vi "destroy_lookup.vi"(8 "error in (no error)":errorcluster, 11 "Mapped Lookup in":refnum<class "Mapped Lookup.lvclass">) -> (0 "error out":errorcluster)   [LabVIEW 2019, in "LVCOOOP.lvlib" / "Lookup API.lvlib" / "Mapped Lookup.lvclass"]
uses:
  Mapped Lookup.lvclass
  Mapped Lookup.lvclass/Mapped Lookup.ctl
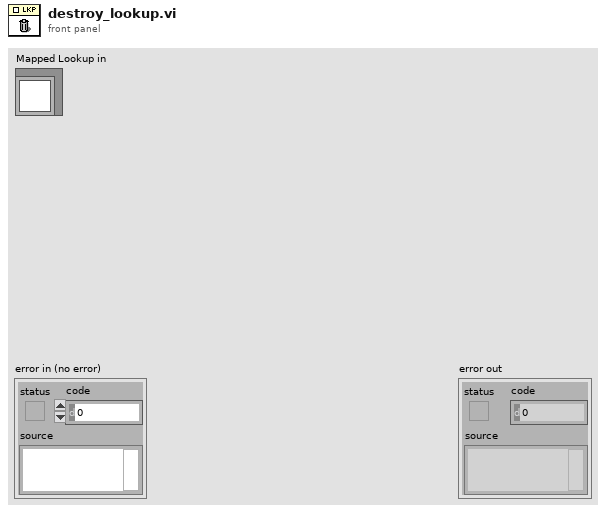
[diagram p1: front panel]
types:
  T1 = map{string, cluster{"instances":refnum<data-value>, "events":refnum<data-value>}}
  T2 = cluster{"instances":refnum<data-value>, "events":refnum<data-value>}
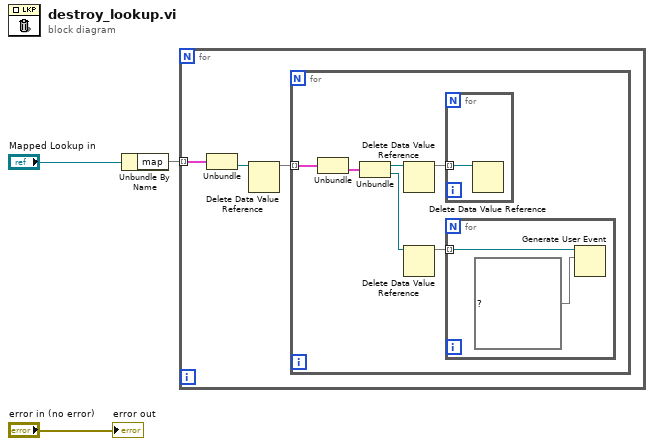
[diagram p0: block diagram]
diagram:
  n1 = Unbundle By Name("Mapped Lookup in") -> ("map"=w2:map{refnum<class>, refnum<data-value>})
  n2 = for {
    tunnel: w2 -> [w6] mode=indexing
    n3 = Unbundle(w6) -> ("named instances"=w5:refnum<data-value>)  [unwired: 1 out]
    n4 = Delete Data Value Reference(data value reference=w5) -> (data value=w4:T1)  [unwired: 1 in, 1 out]
    n5 = for {
      tunnel: w4 -> [w12] mode=indexing
      n6 = Unbundle(w12) -> (w11:T2)  [unwired: 1 out]
      n7 = Unbundle(w11) -> ("instances"=w10:refnum<data-value>, "events"=w9:refnum<data-value>)
      n8 = Delete Data Value Reference(data value reference=w10) -> (data value=w8:set{refnum<data-value>})  [unwired: 1 in, 1 out]
      n9 = Delete Data Value Reference(data value reference=w9) -> (data value=w7:set{refnum<user-event>})  [unwired: 1 in, 1 out]
      n10 = for {
        tunnel: w8 -> [w15] mode=indexing
        n11 = Delete Data Value Reference(data value reference=w15) -> ()  [unwired: 1 in, 2 out]
      }
      n12 = for {
        tunnel: w7 -> [w14] mode=indexing
        n13 = Generate User Event(user event=w14, event data cluster=set{refnum<data-value>} {} ("event data")) -> ()  [unwired: 2 in, 2 out]
      }
    }
  }
  "error out" <- "error in (no error)"
